vi "StringID to Num.vi"(11 "Array":string[](array[string])) -> (3 "Array 2":dbl[](array[numeric]))   [LabVIEW 2015]
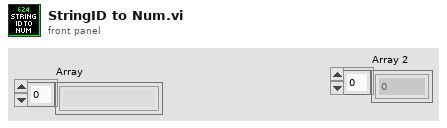
[diagram p1: front panel]
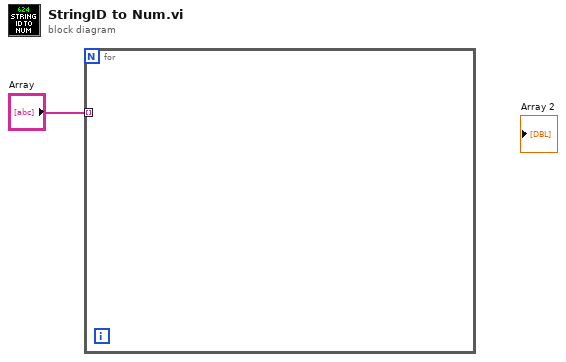
[diagram p0: block diagram]
diagram:
  n1 = for {
    tunnel: "Array" -> [_] mode=indexing
  }
